vi "TBA_NET_Initial.vi"(8 "error in (no error)":errorcluster caption="错误输入（无错误）", 11 "ToolStrip":refnum<k24>(container)) -> (0 "error out":errorcluster caption="错误输出", 2 "User Event":refnum<user-event>, 3 "ToolStrip Out":refnum<class "ToolStrip.lvclass"> caption="Toolbar Ref")   [LabVIEW 2016, in "ToolStrip.lvclass"]
uses:
  Pravite/ToolStrip.lvclass
  Pravite/ToolStrip.lvclass/ToolStrip.ctl
  System.Windows.Forms
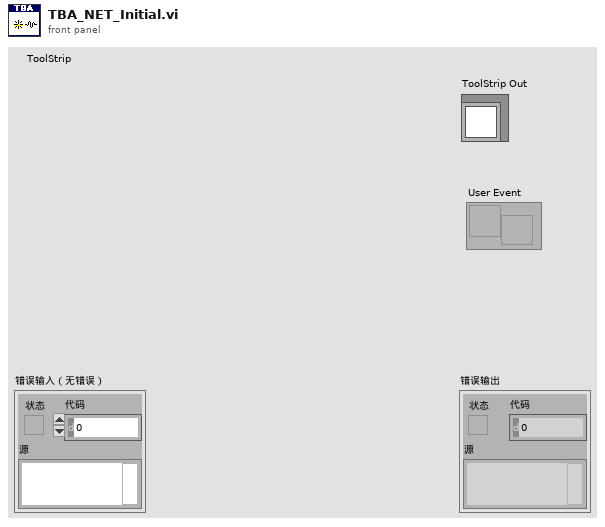
[diagram p1: front panel]
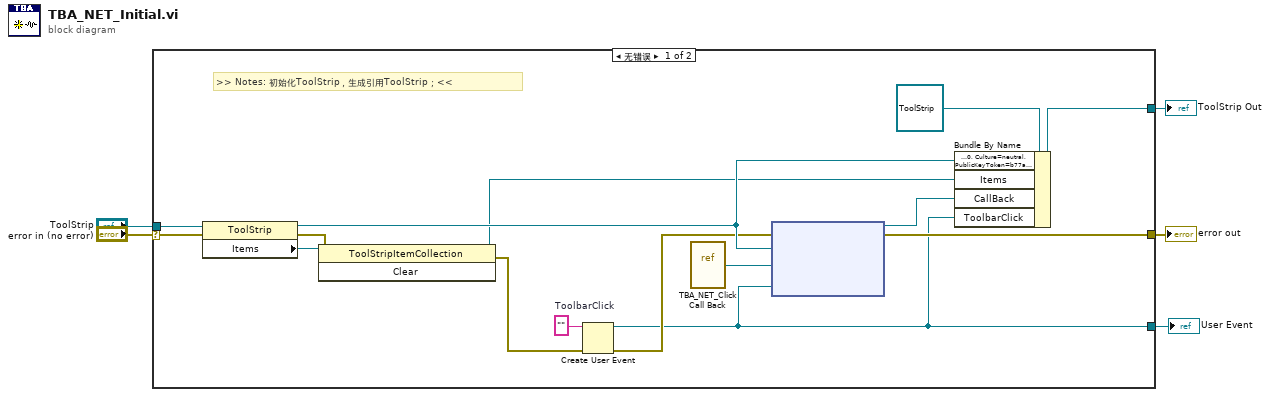
[diagram p0: block diagram]
diagram:
  n1 = case shown="无错误" "error in (no error)" {
    selector: "error in (no error)" -> [w10 w21]
    tunnel: [w9 w21] -> w4
    tunnel: [w6 _] -> w3
    tunnel: "ToolStrip" -> [w11 _]
    tunnel: [w8 _] -> w1
    frame No Error {
      w18 = ""  # ToolbarClick
      # ">> Notes: 初始化ToolStrip，生成引用ToolStrip；<<"
      n2 = property class="ToolStrip"(reference=w11, error in=w10) -> (reference out=w20:refnum<k24>, error out=w15:errorcluster, "Items"=w16:refnum<k24>)
      n3 = invoke class="ToolStripItemCollection" method="Clear"(reference=w16, error in=w15) -> (reference out=w13:refnum<k24>, error out=w14:errorcluster)  [unwired: 1 in, 1 out]
      n4 = Create User Event(user event datatype=w18, error in=w14) -> (user event=w8:refnum<user-event>, error out=w19:errorcluster)
      n5 = vi-ref "TBA_NET_Click Call Back.vi"() -> ("vi reference"=w17:refnum<vi>)
      n6 = node(w19, w20, w17, w8) -> (w12:refnum<k27>, w9:errorcluster)  [unwired: 1 in]
      n7 = Bundle By Name(cluster=refnum<class "ToolStrip.lvclass"> refnum ("ToolStrip 输入"), "ToolStrip"=w20, "Items"=w13, "CallBack"=w12, "ToolbarClick"=w8) -> (w6:refnum<class "ToolStrip.lvclass">)
    }
    frame Error {
    }
  }
  "error out" <- w4
  "ToolStrip Out" <- w3
  "User Event" <- w1
